vi "Clear Scan Time Out_5.vi"(4 "Timeout":i32, 6 "Channel number\nx Sample number":i32, 7 "ESP32 ref":refnum<visa-resource-name>="COM4", 8 "error in (no error)":errorcluster, 11 "VISA Refnum in":refnum<visa-resource-name>) -> (0 "error out":errorcluster, 1 "error?":bool, 2 "Time out count":i32, 3 "VISA Refnum out":refnum<visa-resource-name>, 5 "ESP32 ref out":refnum<visa-resource-name>)   [LabVIEW 2023]
uses:
  <vilib>/Utility/error.llb/DialogType.ctl
  <instrlib>/Agilent 3446X Series/Agilent 3446X Series.lvlib
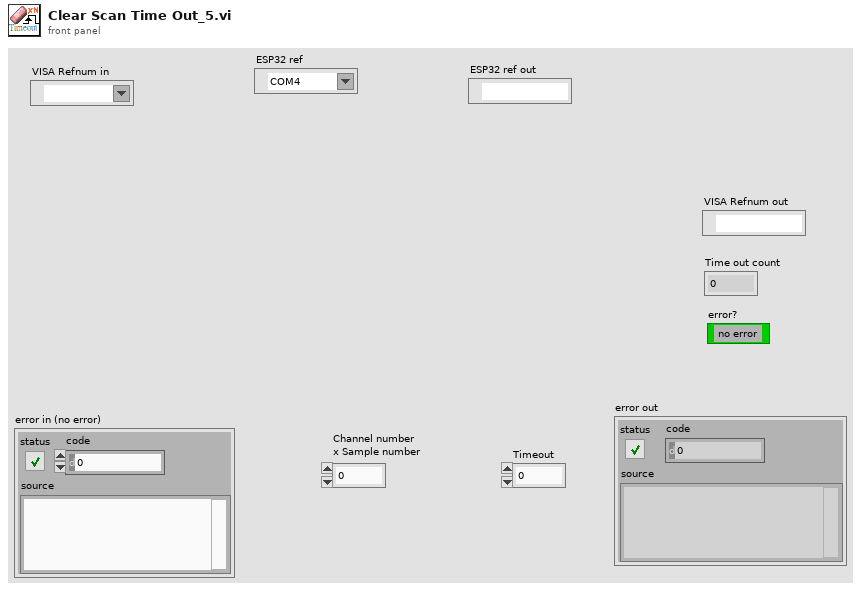
[diagram p1: front panel]
types:
  T1 = typedef "DialogType.ctl" = u16
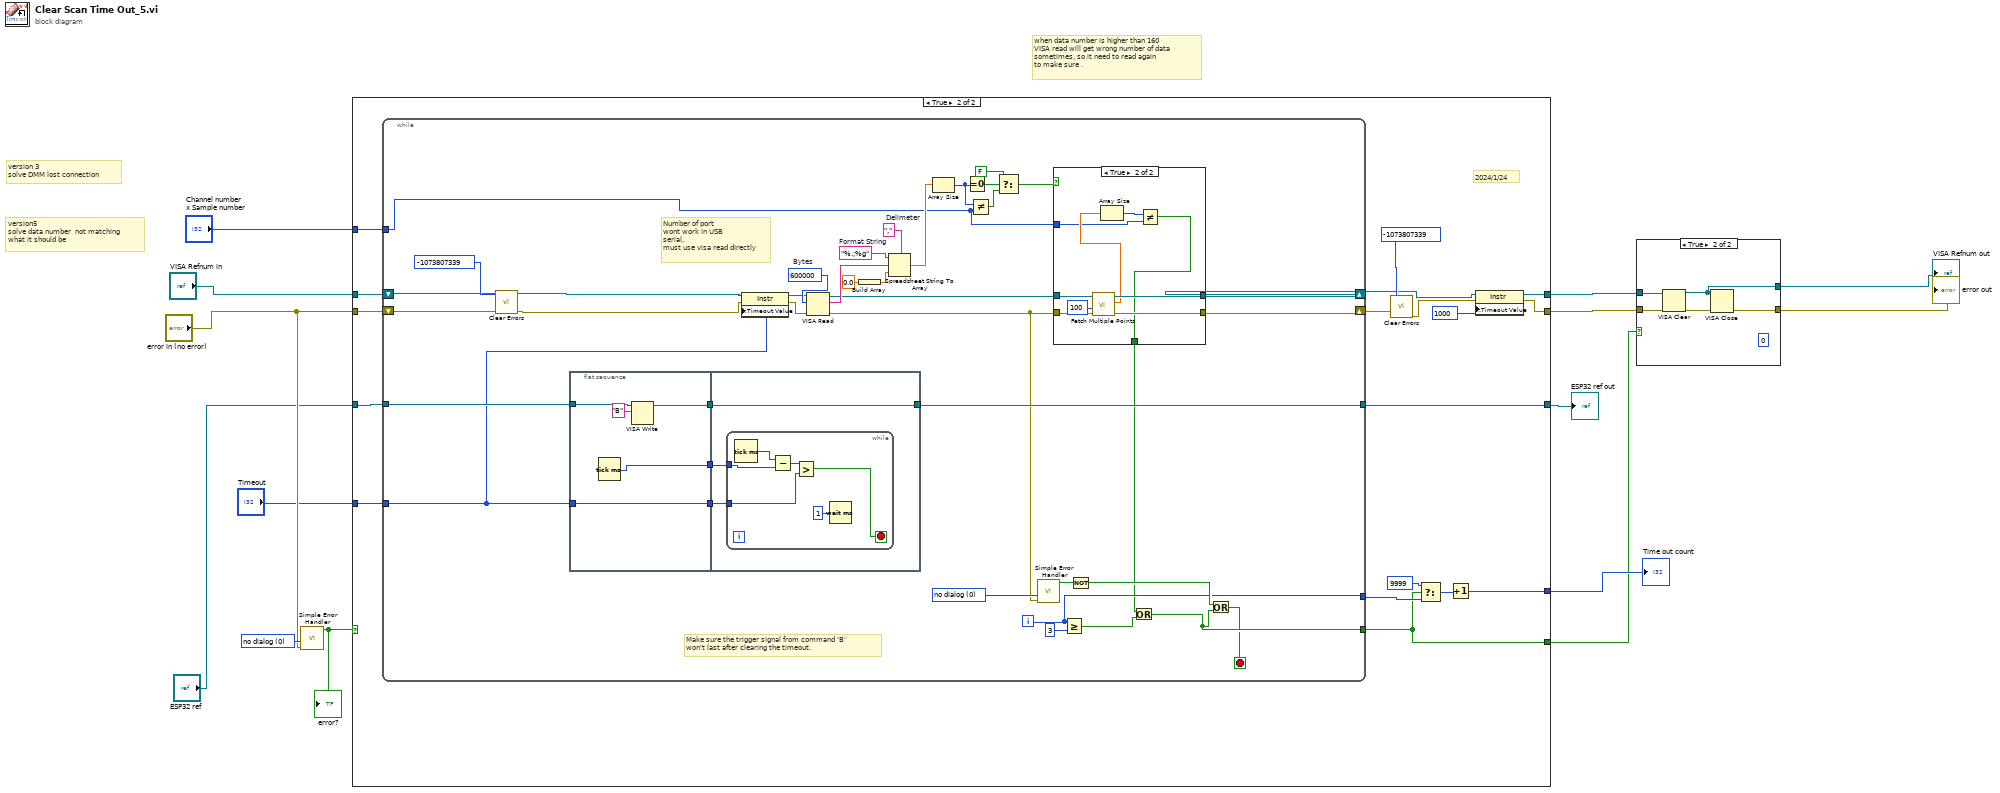
[diagram p0: block diagram]
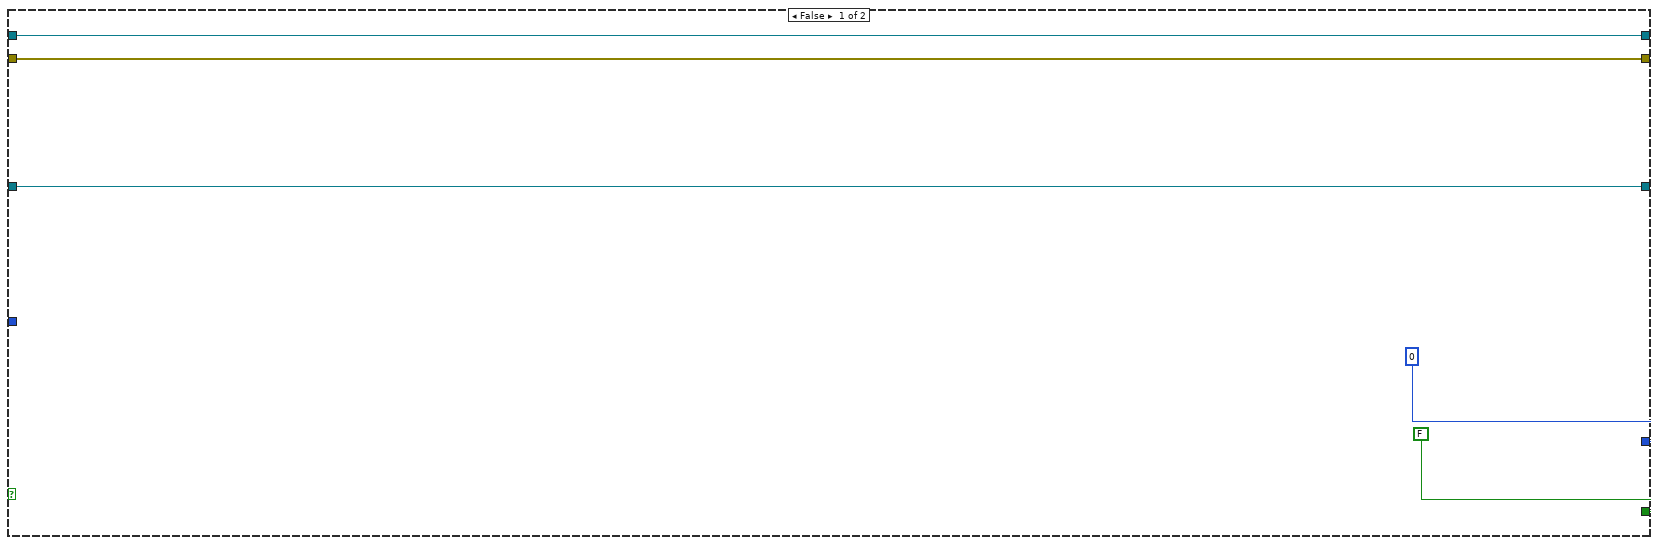
[diagram p3: hidden frame]
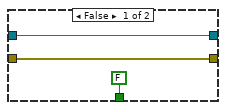
[diagram p4: hidden frame]
diagram:
  w13 = T1 0 items=["no dialog", "OK message", "continue or stop message", "OK message + warnings", "continue/stop + warnings"] ("type of dialog (OK msg:1)")
  # "when data number is higher than 160\nVISA read will get wrong number of data\nsometimes, so it need to read again\nto make sure ."
  # "version5\nsolve data number  not matching\nwhat it should be"
  # "version 3\nsolve DMM lost connection"
  n1 = call <vilib>:"Simple Error Handler.vi"("type of dialog (OK msg:1)"=w13, "error in (no error)"="error in (no error)") -> ("error?"=w11:bool)  [unwired: 3 in, 4 out]
  "error?" <- w11
  n2 = case shown="True" w11 {
    tunnel: [w19 w20] -> w5
    tunnel: "error in (no error)" -> [w18 w37]
    tunnel: "VISA Refnum in" -> [w19 w36]
    tunnel: [w18 w21] -> w4
    tunnel: [0 w35] -> w10
    tunnel: "ESP32 ref" -> [w17 w33]
    tunnel: [w17 w32] -> w8
    tunnel: "Channel number\nx Sample number" -> [_ w31]
    tunnel: [FALSE w26] -> w6
    tunnel: "Timeout" -> [_ w25]
    frame False {
    }
    frame True {
      # "2024/1/24"
      n3 = while {
        shift-right: [w42] -> w30
        shift-left: w37 -> [w74]
        shift-right: [w43] -> w22
        shift-left: w36 -> [w60]
        tunnel: [w49] -> w27
        tunnel: [w56] -> w26
        tunnel: w33 -> [w59]
        tunnel: [w51] -> w32
        tunnel: w31 -> [w44]
        tunnel: w25 -> [w38]
        i -> [w49]
        stop <- w50 stop-if-true
        w67 = ","  # Delimeter
        w68 = "%.;%g"  # Format String
        w63 = u32 600000  # Bytes
        w72 = T1 0 items=["no dialog", "OK message", "continue or stop message", "OK message + warnings", "continue/stop + warnings"] ("type of dialog (OK msg:1)")
        # "Make sure the trigger signal from command 'B' \nwon't last after clearing the timeout."
        # "Number of port\nwont work in USB \nserial,\nmust use visa read directly"
        n4 = call <vilib>:"Clear Errors.vi"("error in (no error)"=w74, "specific error code to clear (0: all)"=-1073807339 ("code out")) -> ("error out"=w73:errorcluster)  [unwired: 4 in, 1 out]
        n5 = flat-sequence {
          tunnel: w59 -> [w79]
          tunnel: [w78] -> w41
          tunnel: [w77] -> w40
          tunnel: w38 -> [w76]
          tunnel: [w76] -> w39
          tunnel: [w83] -> w51
          tunnel: w41 -> [w83]
          tunnel: w40 -> [w82]
          tunnel: w39 -> [w81]
          frame #0 {
            n6 = Tick Count (ms)() -> (millisecond timer value=w77:u32)
            n7 = VISA Write(VISA resource name=w79, write buffer="B") -> (VISA resource name out=w78:refnum<visa-resource-name>)  [unwired: 1 in, 2 out]
          }
          frame #1 {
            n8 = while {
              tunnel: w82 -> [w88]
              tunnel: w81 -> [w86]
              stop <- w84 stop-if-true
              n9 = Tick Count (ms)() -> (millisecond timer value=w89:u32)
              n10 = Subtract(x=w89, y=w88) -> (x-y=w87:u32)
              n11 = Greater?(x=w87, y=w86) -> (0:w84:bool)
              n12 = Wait (ms)(milliseconds to wait=u32 1) -> ()  [unwired: 1 out]
            }
          }
        }
        n13 = property class="Instr"(reference=w60, error in=w73, "General Settings:Timeout Value"=w38) -> (reference out=w62:refnum<visa-resource-name>, error out=w61:errorcluster)
        n14 = VISA Read(VISA resource name=w62, byte count=w63, error in (no error)=w61) -> (VISA resource name out=w47:refnum<visa-resource-name>, read buffer=w64:string, error out=w46:errorcluster)  [unwired: 1 out]
        n15 = Build Array(0.0) -> (w65:dbl[])
        n16 = Spreadsheet String To Array(delimiter (Tab)=w67, format string=w68, spreadsheet string=w64, array type (2D Dbl)=w65) -> (array=w58:dbl[])
        n17 = Array Size(array=w58) -> (size(s)=w52:i32)
        n18 = Equal To 0?(x=w52) -> (x = 0?=w55:bool)
        n19 = Not Equal?(x=w52, y=w44) -> (x != y?=w54:bool)
        n20 = Select(t=FALSE, s=w55, f=w54) -> (s? t:f=w48:bool)
        n21 = call <vilib>:"Simple Error Handler.vi"("type of dialog (OK msg:1)"=w72, "error in (no error)"=w46) -> ("error?"=w69:bool)  [unwired: 3 in, 4 out]
        n22 = case shown="True" w48 {
          tunnel: w47 -> [w92 w101]
          tunnel: w46 -> [w91 w100]
          tunnel: [w92 w98] -> w43
          tunnel: [w91 w97] -> w42
          tunnel: [FALSE ("t") w94] -> w45
          tunnel: w44 -> [_ w93]
          frame False {
          }
          frame True {
            n23 = call <instrlib>:"Fetch Multiple Points.vi"("error in (no error)"=w100, "Timeout (10000 ms)"=100, "VISA resource name"=w101) -> ("error out"=w97:errorcluster, "Measurements"=w95:dbl[], "VISA resource name out"=w98:refnum<visa-resource-name>)  [unwired: 6 in]
            n24 = Array Size(array=w95) -> (size(s)=w96:i32)
            n25 = Not Equal?(x=w96, y=w93) -> (x != y?=w94:bool)
          }
        }
        n26 = Greater Or Equal?(x=w49, y=3) -> (x >= y?=w57:bool)
        n27 = Not(x=w69) -> (.not. x?=w70:bool)
        n28 = Or(x=w45, y=w57) -> (x .or. y?=w56:bool)
        n29 = Or(x=w70, y=w56) -> (x .or. y?=w50:bool)
      }
      n30 = call <vilib>:"Clear Errors.vi"("error in (no error)"=w30, "specific error code to clear (0: all)"=-1073807339 ("code out")) -> ("error out"=w23:errorcluster)  [unwired: 4 in, 1 out]
      n31 = Select(t=9999, s=w26, f=w27) -> (s? t:f=w34:i32)
      n32 = Increment(x=w34) -> (x+1=w35:i32)
      n33 = property class="Instr"(reference=w22, error in=w23, "General Settings:Timeout Value"=u32 1000) -> (reference out=w20:refnum<visa-resource-name>, error out=w21:errorcluster)
    }
  }
  "Time out count" <- w10
  "ESP32 ref out" <- w8
  n34 = case shown="True" w6 {
    tunnel: w5 -> [w103 w107]
    tunnel: w4 -> [w102 w108]
    tunnel: [w102 w105] -> w3
    tunnel: [w103 w104] -> w2
    frame False {
    }
    frame True {
      (unwired) u32 0
      n35 = VISA Clear(VISA resource name=w107, error in (no error)=w108) -> (VISA resource name out=w104:refnum<visa-resource-name>, error out=w106:errorcluster)
      n36 = VISA Close(VISA resource name=w104, error in (no error)=w106) -> (error out=w105:errorcluster)
    }
  }
  "error out" <- w3
  "VISA Refnum out" <- w2
